vi "subviexo3.vi"(11 "degré":dbl) -> (0 "LED3":bool, 1 "LED2":bool, 2 "LED1":bool, 3 "LED0":bool)   [LabVIEW 2019]
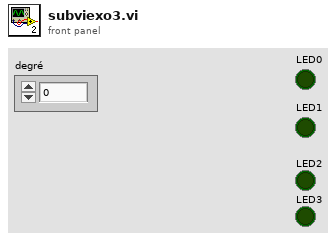
[diagram p1: front panel]
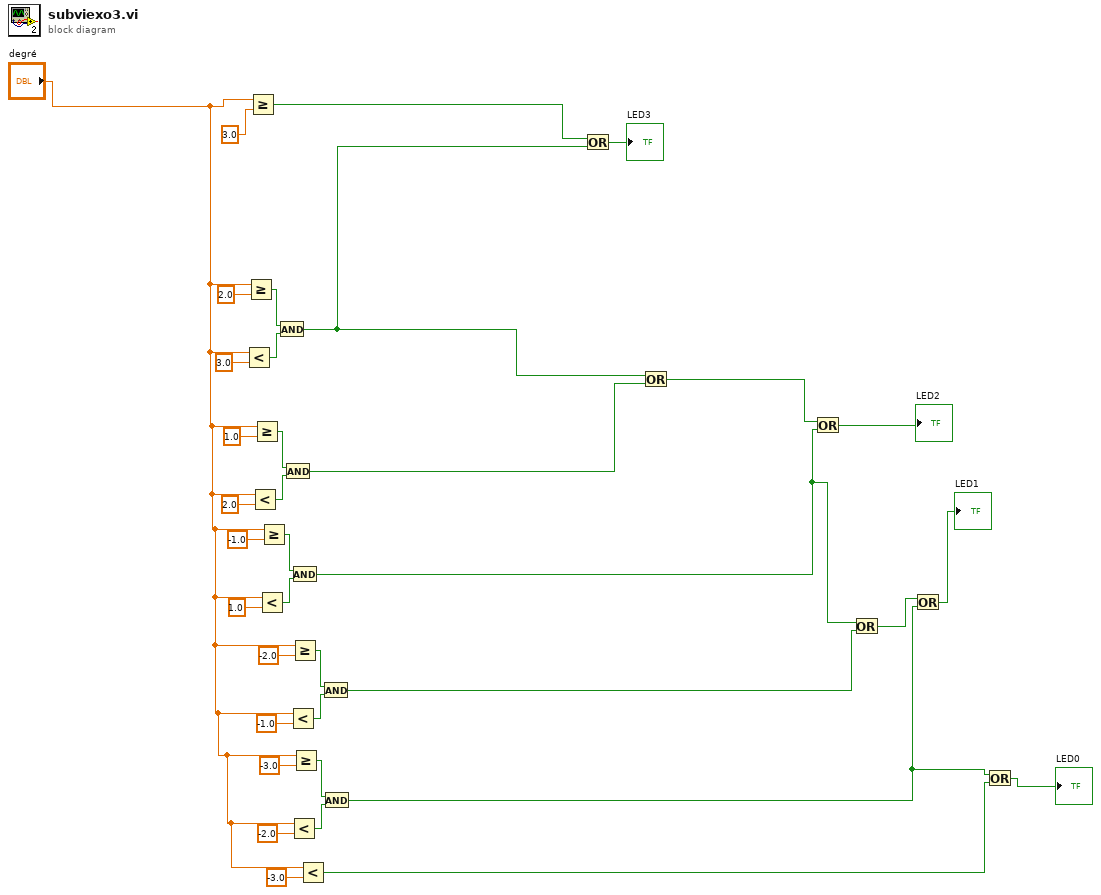
[diagram p0: block diagram]
diagram:
  n1 = Less?(x="degré", y=3.0) -> (x < y?=w6:bool)
  n2 = Greater Or Equal?(x="degré", y=2.0) -> (x >= y?=w5:bool)
  n3 = Greater Or Equal?(x="degré", y=3.0) -> (x >= y?=w7:bool)
  n4 = Less?(x="degré", y=2.0) -> (x < y?=w12:bool)
  n5 = Greater Or Equal?(x="degré", y=1.0) -> (x >= y?=w11:bool)
  n6 = Less?(x="degré", y=1.0) -> (x < y?=w17:bool)
  n7 = Greater Or Equal?(x="degré", y=-1.0) -> (x >= y?=w16:bool)
  n8 = And(x=w5, y=w6) -> (x .and. y?=w18:bool)
  n9 = And(x=w11, y=w12) -> (x .and. y?=w13:bool)
  n10 = Less?(x="degré", y=-1.0) -> (x < y?=w25:bool)
  n11 = Less?(x="degré", y=-2.0) -> (x < y?=w30:bool)
  n12 = And(x=w16, y=w17) -> (x .and. y?=w21:bool)
  n13 = Greater Or Equal?(x="degré", y=-2.0) -> (x >= y?=w24:bool)
  n14 = Greater Or Equal?(x="degré", y=-3.0) -> (x >= y?=w29:bool)
  n15 = Less?(x="degré", y=-3.0) -> (x < y?=w35:bool)
  n16 = And(x=w24, y=w25) -> (x .and. y?=w26:bool)
  n17 = And(x=w29, y=w30) -> (x .and. y?=w34:bool)
  n18 = Or(x=w7, y=w18) -> (x .or. y?=→"LED3":bool)
  n19 = Or(x=w18, y=w13) -> (x .or. y?=w19:bool)
  n20 = Or(x=w19, y=w21) -> (x .or. y?=→"LED2":bool)
  n21 = Or(x=w21, y=w26) -> (x .or. y?=w31:bool)
  n22 = Or(x=w31, y=w34) -> (x .or. y?=→"LED1":bool)
  n23 = Or(x=w34, y=w35) -> (x .or. y?=→"LED0":bool)
